vi "Set started from.vi"(8 "error in (no error)":errorcluster, 10 "started by tomo?":bool, 11 "ImageStack in":refnum<class "ImageStack.lvclass">) -> (0 "error out":errorcluster, 3 "ImageStack out":refnum<class "ImageStack.lvclass">)   [LabVIEW 2012, in "ImageStack.lvclass"]
uses:
  ImageStack.lvclass
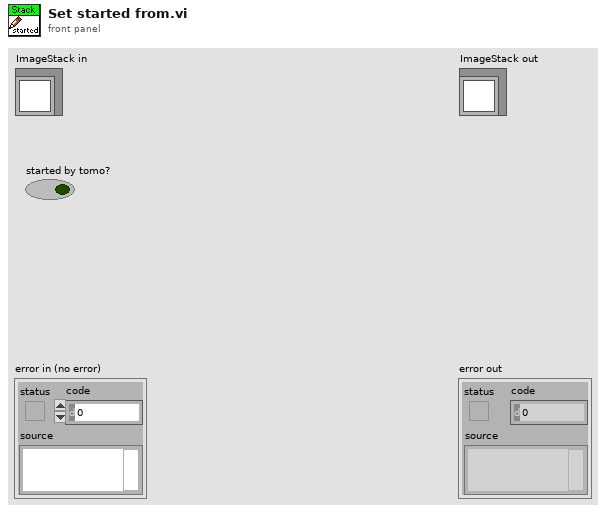
[diagram p1: front panel]
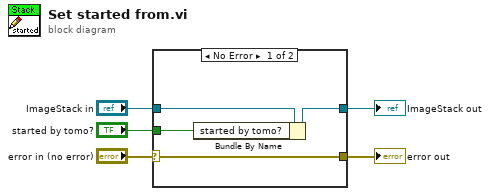
[diagram p0: block diagram]
diagram:
  n1 = case shown="No Error" "error in (no error)" {
    selector: "error in (no error)" -> [w9 w11]
    tunnel: [w9 w11] -> w4
    tunnel: [w7 w10] -> w2
    tunnel: "ImageStack in" -> [w8 w10]
    tunnel: "started by tomo?" -> [w6 _]
    frame No Error {
      n2 = Bundle By Name(cluster=w8, "started by tomo?"=w6) -> (w7:refnum<class "ImageStack.lvclass">)
    }
    frame Error {
    }
  }
  "error out" <- w4
  "ImageStack out" <- w2
